vi "Standard_Function_gen.vi"(0 "Instrument handle in":refnum<k15>, 1 "Channel name":string, 2 "User defined waveform":dbl[](array[numeric]) format="%.2f", 3 "Waveform":T1(ring), 5 "Trigger mode":u32, 7 "Trigger source":u32, 9 "Amplitude":dbl format="%.2f", 11 "error in (no error)":errorcluster, 12 "DC Offset":dbl format="%.2f", 13 "Start phase":dbl format="%.2f", 14 "Frequency":dbl format="%.2f") -> (4 "Instrument handle out":refnum<k15>, 15 "error out":errorcluster)   [LabVIEW 2011]
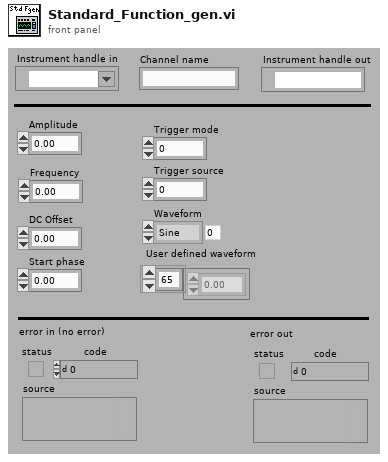
[diagram p1: front panel]
types:
  T1 = enum16{"Sine", "Square", "Triangle", "Ramp up", "Ramp down", "DC", "Noise", "User Defined"}
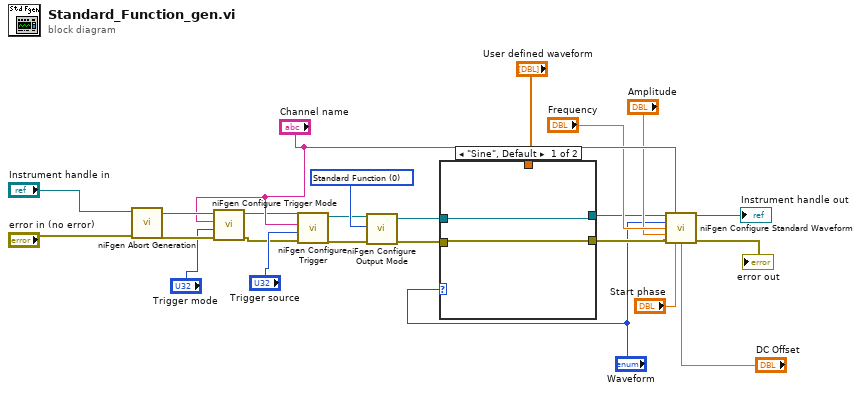
[diagram p0: block diagram]
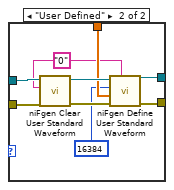
[diagram p2: hidden frame]
diagram:
  w20 = u32 0 items=["Standard Function", "Frequency List", "Arbitrary Waveform", "Arbitrary Sequence"] ("output mode")
  n1 = call <instrlib>:"niFgen Abort Generation.vi"("error in (no error)"="error in (no error)", "Instrument Handle"="Instrument handle in") -> ("error out"=w23:errorcluster, "Instrument Handle Out"=w24:refnum<k15>)  [unwired: 8 in]
  n2 = call <instrlib>:"niFgen Configure Trigger Mode.vi"("error in (no error)"=w23, "Trigger Mode (default: 1=continuous)"="Trigger mode", "Channel Name"="Channel name", "Instrument Handle"=w24) -> ("error out"=w10:errorcluster, "Instrument Handle Out"=w9:refnum<k15>)  [unwired: 6 in]
  n3 = call <instrlib>:"niFgen Configure Trigger.vi"("error in (no error)"=w10, "Trigger Source (default: 0=immediate)"="Trigger source", "Channel Name"="Channel name", "Instrument Handle"=w9) -> ("error out"=w17:errorcluster, "Instrument Handle Out"=w16:refnum<k15>)  [unwired: 6 in]
  n4 = call <instrlib>:"niFgen Configure Output Mode.vi"("error in (no error)"=w17, "Output Mode (default: 0=Standard Function)"=w20, "Instrument Handle"=w16) -> ("error out"=w18:errorcluster, "Instrument Handle Out"=w19:refnum<k15>)  [unwired: 6 in]
  n5 = case shown="\"Sine\", Default" "Waveform" {
    tunnel: w18 -> [w25 w35]
    tunnel: w19 -> [w26 w34]
    tunnel: [w25 w31] -> w8
    tunnel: [w26 w30] -> w2
    tunnel: "User defined waveform" -> [_ w29]
    frame "Sine", Default {
    }
    frame "User Defined" {
      w28 = "0"
      n6 = call <instrlib>:"niFgen Clear User Standard Waveform.vi"("error in (no error)"=w35, "Channel Name"=w28, "Instrument Handle"=w34) -> ("error out"=w32:errorcluster, "Instrument Handle Out"=w33:refnum<k15>)  [unwired: 7 in]
      n7 = call <instrlib>:"niFgen Define User Standard Waveform.vi"("Channel Name"=w28, "error in (no error)"=w32, "Waveform Data Array"=w29, "Waveform Size"=16384, "Instrument Handle"=w33) -> ("error out"=w31:errorcluster, "Instrument Handle Out"=w30:refnum<k15>)  [unwired: 5 in]
    }
  }
  n8 = call <instrlib>:"niFgen Configure Standard Waveform.vi"("Instrument Handle"=w2, "Channel Name"="Channel name", "Waveform"="Waveform", "Frequency"="Frequency", "Amplitude"="Amplitude", "error in (no error)"=w8, "Start Phase"="Start phase", "DC Offset"="DC Offset") -> ("Instrument Handle Out"=→"Instrument handle out":refnum<k15>, "error out"=→"error out":errorcluster)  [unwired: 6 in]
